vi "SCH Protection-RT Host.vi"() -> ()   [LabVIEW 2020]
doc: "Author: Scott Hannahs <sth@magnet.fsu.edu>\nCopyright 2018 Florida State University, All rights reserved."
uses:
  <vilib>/Platform/TimedLoop/XDataNode/timing_clust.ctl
  <vilib>/Platform/TimedLoop/XDataNode/nitl_modes.ctl
  <vilib>/Platform/TimedLoop/XDataNode/wakeup.ctl
  RT Server Sub VIs/RT Host Globals.vi
  <vilib>/Utility/error.llb/Error Cluster From Error Code.vi
  <vilib>/rvi/errors/niLvFpgaAdjustHostInterfaceError.vi
  <vilib>/functionblocks/Edge Detection/One Shot Falling With Input/One Shot Falling With Input.vi
  <vilib>/rvi/interface/nirviReadWriteControl/nirviReadWriteControl.xnode
  RT Controls/FPGA SCH Digitizer Ref.ctl
  <vilib>/functionblocks/FB Core/FB Core.xnode
  <vilib>/Platform/TimedLoop/XDataNode/XDataNode.xnode
  <vilib>/functionblocks/NI_FunctionBlock Libraries.lvlib
  <vilib>/NI_Real-Time Target Support.lvlib
  NiFpgaLv.dll
  <vilib>/rvi/interface/Simulation/niFpgaSimulationCallBeginRW.vi
  <vilib>/Platform/TimedLoop/XDataNode/XDNodeRunTimeDep.lvlib
panel:
  out "Finished Late?":bool
  out "Iteration Duration (microS)":i64
  in  "Data Logging Time (mS)":u32=1000
  in  "Build":u8=115
  in  "Fix":u8=2
  in  "Minor":u8=9
  in  "Major":u8=2
  out "# Network Connections":i32
  out "Error Out Connection Loop":errorcluster
  out "Mismatch":bool
  out "Error Out FIFO Loop":errorcluster
  out "#Data sets":u32
  out "Total Data Sets":u64
  out "Reading Rate":dbl format="%.1f"
  # "SCH Protection Real Time System"
  # "."
  # "."
  # "."
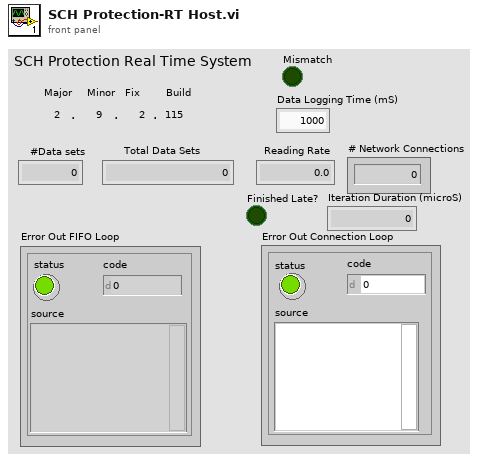
[diagram p1: front panel]
types:
  T1 = typedef "FPGA SCH Digitizer Ref.ctl" = refnum<k20>
  T2 = typedef "Net Conn Handler VI.ctl" = refnum<vi>
  T3 = typedef "XDNodeRunTimeDep.lvlib/timing_clust.ctl" = cluster{"Expected End [f-1]":u64, "Actual End [f-1]":u64, "Finished Late? [f-1]":bool, "Expected End [i-1]":u64, "Actual End [i-1]":u64, "Finished Late? [i-1]":bool, "Expected Start [i]":u64, "Actual Start [i]":u64, "Expected Start [f]":u64, "Actual Start [f]":u64, "Source Name":string, "Structure Name":string, "Period":i64, "Deadline":i64, "Offset":i64, "Start":i64, "Priority":i32, "Timeout":i32, "Mode":T4, "Wakeup Reason":T5, "Error":errorcluster, "Source Type":string, "Secondary Source Type":string, "Global End Time":u64, "Global Start Time":u64, "Frame Duration":u64, "Iteration Duration":u64, "Assigned CPU":i32, "I/O Scan Engine Mode":u32}
  T4 = typedef "XDNodeRunTimeDep.lvlib/nitl_modes.ctl" = enum32{"No Change", "Process missed periods, maintain original phase", "Discard missed periods, maintain original phase", "Process missed periods, ignore original phase", "Discard missed periods, ignore original phase"}
  T5 = typedef "XDNodeRunTimeDep.lvlib/wakeup.ctl" = enum32{"Normal", "Aborted", "Asynchronous wakeup", "Timing source error", "Timed loop error", "Timeout"}
  T6 = enum16{"Input Voltage", "Zero Voltage", "Calibrate Voltage"}
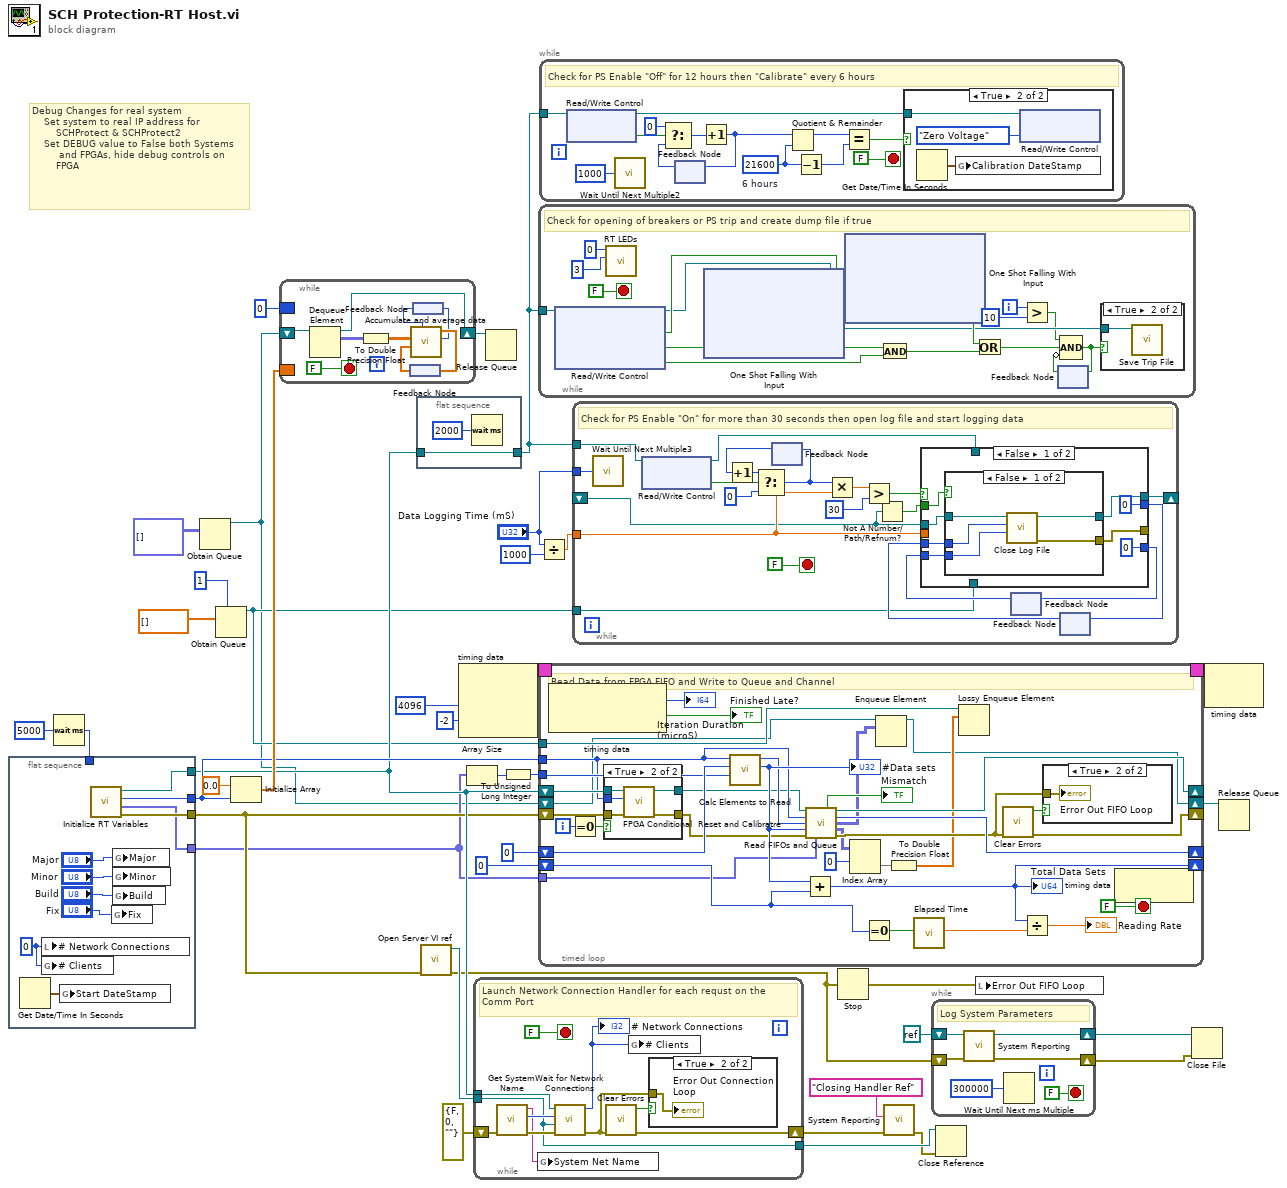
[diagram p0: block diagram]
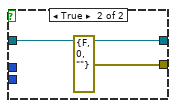
[diagram p5: hidden frame]
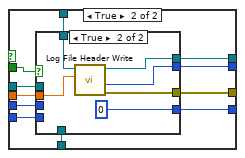
[diagram p6: hidden frame]
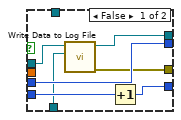
[diagram p7: hidden frame]
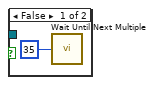
[diagram p8: hidden frame]
diagram:
  # "Debug Changes for real system\n    Set system to real IP address for\n        SCHProtect & SCHProtect2\n    Set DEBUG value to False both Systems\n         and FPGAs, hide debug controls on\n        FPGA"
  n1 = flat-sequence {
    tunnel: [w48] -> w34
    tunnel: [w47] -> w28
    tunnel: [w46] -> w30
    tunnel: w24 -> [_]
    tunnel: [w41] -> w15
    frame #0 {
      w40 = 0 ("# Connections")
      n2 = Get Date/Time In Seconds() -> (seconds since 1Jan1904=w39:timestamp)
      n3 = local write "# Network Connections"(w40) -> ()
      n4 = global write "RT Host Globals.vi" "# Clients"(w40) -> ()
      n5 = global write "RT Host Globals.vi" "Start DateStamp"(w39) -> ()
      n6 = call "Initialize RT Variables.vi"() -> ("error out"=w47:errorcluster, "Sync Guard Data"=w41:fxp<+/-,38,12>[], "Data Size"=w48:u32, "FPGA Refnum out"=w46:T1)  [unwired: 8 in]
      n7 = global write "RT Host Globals.vi" "Fix"("Fix") -> ()
      n8 = global write "RT Host Globals.vi" "Major"("Major") -> ()
      n9 = global write "RT Host Globals.vi" "Minor"("Minor") -> ()
      n10 = global write "RT Host Globals.vi" "Build"("Build") -> ()
    }
  }
  n11 = Wait (ms)(milliseconds to wait=u32 5000) -> (millisecond timer value=w24:u32)
  n12 = Obtain Queue(element data type=fxp<+/-,38,12>[][] [] ("Data Unfiltered")) -> (queue out=w3:refnum<queue>)  [unwired: 4 in, 2 out]
  n13 = Obtain Queue(max queue size (-1, unlimited)=1, element data type=dbl[] [] ("double precision float")) -> (queue out=w5:refnum<queue>)  [unwired: 3 in, 2 out]
  n14 = Initialize Array(0.0, w34) -> (w36:dbl[])
  n15 = while {
    border: w36 -> [_]
    border: 0 -> [_]
    shift-right: [w49] -> w2
    shift-left: w3 -> [w50]
    stop <- FALSE stop-if-true
    n16 = Dequeue Element(queue=w50) -> (queue out=w49:refnum<queue>, element=w51:fxp<+/-,38,12>[][])  [unwired: 2 in, 2 out]
    n17 = To Double Precision Float(number=w51) -> (double precision float=w52:dbl[][])
    n18 = feedback #1() -> (w57:dbl[])
    n19 = feedback #2() -> (w53:i32)
    n20 = call "Accumulate and average data.vi"("# Scans Accululated In"=w53, "Accumulated Array"=w57, "Raw Data In"=w52) -> ("# Scans Accumulated Out"=w54:i32, "Accumulated Array Out"=w56:dbl[])  [unwired: 7 in]
    n21 = feedback-in #1(w56) -> ()
    n22 = feedback-in #2(w54) -> ()
  }
  n23 = flat-sequence {
    tunnel: w30 -> [w59]
    tunnel: [w59] -> w33
    frame #0 {
      n24 = Wait (ms)(milliseconds to wait=u32 2000) -> ()  [unwired: 1 out]
    }
  }
  n25 = call "Open Server VI ref.vi"("error in (no error)"=w28) -> ("error out"=w12:errorcluster, "VI out"=w22:T2)  [unwired: 9 in]
  n26 = node-c288(i64 4096 ("Period"), -2 ("Processor")) -> (w17:T3)  [unwired: 1 in]
  n27 = Array Size(array=w15) -> (size(s)=w14:i32)
  n28 = while {
    shift-right: [w68] -> w20
    shift-left: errorcluster {"status"=FALSE, "code"=0, "source"=""} ("Error Out") -> [w64]
    tunnel: w30 -> [w66]
    tunnel: w22 -> [w62]
    tunnel: [w62] -> w21
    stop <- FALSE stop-if-true
    # "Launch Network Connection Handler for each requst on the Comm Port"
    n29 = call "Get System Name.vi"("Error In"=w64) -> ("Error Out"=w63:errorcluster, "Ethernet Address"=w65:u32, "System Name"=w60:string)  [unwired: 4 in]
    n30 = global write "RT Host Globals.vi" "System Net Name"(w60) -> ()
    n31 = call "Wait for Network Connections.vi"("error in (no error)"=w63, "Handler VI ref"=w62, "Ethernet Address"=w65, "FPGA Refnum in"=w66) -> ("error out"=w69:errorcluster, "# Network Connections"=w61:i32)  [unwired: 6 in]
    "# Network Connections" <- w61
    n32 = call <vilib>:"Clear Errors.vi"("error in (no error)"=w69) -> ("error out"=w68:errorcluster, "specific error cleared?"=w67:bool)  [unwired: 5 in]
    n33 = global write "RT Host Globals.vi" "# Clients"(w61) -> ()
    n34 = case shown="True" w67 {
      tunnel: w69 -> [_ w71]
      frame False {
      }
      frame True {
        "Error Out Connection Loop" <- w71
      }
    }
  }
  n35 = Release Queue(queue=w2) -> ()  [unwired: 2 in, 3 out]
  n36 = To Unsigned Long Integer(number=w14) -> (unsigned 32bit integer=w13:u32)
  n37 = while {
    tunnel: w33 -> [w87]
    i -> [w75]
    stop <- FALSE stop-if-true
    # "Check for opening of breakers or PS trip and create dump file if true"
    n38 = xnode "Read/Write Control"("FPGA VI Reference In"=w87) -> ("FPGA VI Reference Out"=w77:T1, "Breaker Enable"=w86:bool, "PS Enable"=w85:bool, "Dump File Enable"=w83:bool)  [unwired: 1 in, 1 out]
    n39 = call <vilib>:"RT LEDs.vi"("State"=3, "LED Num"=0) -> ()  [unwired: 4 in, 2 out]
    n40 = xnode "One Shot Falling With Input"("input"=w85) -> ("output"=w84:bool)  [unwired: 1 in, 1 out]
    n41 = xnode "One Shot Falling With Input"("input"=w86) -> ("output"=w82:bool)  [unwired: 1 in, 1 out]
    n42 = And(x=w84, y=w83) -> (x .and. y?=w81:bool)
    n43 = Or(x=w82, y=w81) -> (x .or. y?=w80:bool)
    n44 = Greater?(x=w75, y=10) -> (0:w76:bool)
    n45 = feedback #3() -> (w73:bool)  [unwired: 1 in]
    n46 = Compound Arithmetic op=AND(w76, w80, invert w73) -> (w72:bool)
    n47 = feedback-in #3(w72) -> ()
    n48 = case shown="True" w72 {
      tunnel: w77 -> [_ w90]
      frame False {
        n49 = call "Wait Until Next Multiple"("Count(mSec)"=u32 35) -> ()  [unwired: 1 out]
      }
      frame True {
        n50 = call "Save Trip File.vi"("FPGA Refnum"=w90) -> ()  [unwired: 10 in, 1 out]
      }
    }
  }
  n51 = Divide(x="Data Logging Time (mS)", y=u32 1000) -> (x/y=w32:dbl)
  n52 = timed-loop {
    shift-right: [w195] -> _
    shift-left: u32 0 -> [w198]
    tunnel: w34 -> [w175]
    shift-right: [w194] -> _
    shift-left: u64 0 -> [w197]
    shift-right: [w190] -> _
    shift-left: w30 -> [w178]
    shift-right: [w187] -> _
    shift-left: w28 -> [w177]
    timing: w17 -> [_]
    timing-out: [_] -> w16
    tunnel: w15 -> [w182]
    tunnel: w13 -> [w181]
    tunnel: w5 -> [w170]
    shift-right: [w167] -> w1
    shift-left: w3 -> [w168]
    i -> [w180]
    stop <- FALSE stop-if-true
    # "Read Data from FPGA FIFO and Write to Queue and Channel"
    n53 = node-c288() -> (→"Iteration Duration (microS)":i64, →"Finished Late?":bool)  [unwired: 1 in]
    n54 = Equal To 0?(x=w180) -> (x = 0?=w179:bool)
    n55 = case shown="True" w179 {
      tunnel: w178 -> [w202 w207]
      tunnel: [w202 w206] -> w172
      tunnel: [w201 w205] -> w176
      tunnel: w177 -> [w201 w204]
      tunnel: w175 -> [_ w203]
      frame False {
      }
      frame True {
        n56 = call "FPGA Conditional  Reset and Calibratre.vi"("error in (no error)"=w204, "Data Size"=w203, "Refnum in"=w207) -> ("error out"=w205:errorcluster, "Refnum out"=w206:T1)  [unwired: 6 in, 1 out]
      }
    }
    n57 = call "Calc Elements to Read.vi"("Sync Guard Data Length"=w181, "Elements in FIFO"=w198, "Data Size"=w175) -> ("# Data Sets To Read"=w192:u32, "# Elements to Read"=w188:u32)  [unwired: 7 in]
    "#Data sets" <- w192
    n58 = Add(x=w192, y=w197) -> (x+y=w194:u64)
    "Total Data Sets" <- w194
    n59 = call "Read FIFOs and Queue.vi"("FPGA VI Reference"=w172, "Data Size"=w175, "# Elements to Read"=w188, "# Data Sets To Read"=w192, "error in (no error)"=w176, "Sync Guard Data"=w182) -> ("Read Mismatch"=→"Mismatch":bool, "Refnum out"=w190:T1, "Elements Remaining"=w195:u32, "Data Unfiltered"=w169:fxp<+/-,38,12>[][], "DataFiltered"=w184:fxp<+/-,38,12>[][], "error out"=w189:errorcluster)  [unwired: 4 in]
    n60 = Index Array(array=w184, index (row)=0 ("index")) -> (element=w183:fxp<+/-,38,12>[])  [unwired: 1 in]
    n61 = Equal To 0?(x=w197) -> (x = 0?=w199:bool)
    n62 = Enqueue Element(queue=w168, element=w169) -> (queue out=w167:refnum<queue>)  [unwired: 2 in, 2 out]
    n63 = To Double Precision Float(number=w183) -> (double precision float=w171:dbl[])
    n64 = call "Elapsed Time"("Reset"=w199) -> ("Elapsed Time (s)"=w200:dbl)  [unwired: 11 in, 7 out]
    n65 = Lossy Enqueue Element(queue=w170, element=w171) -> ()  [unwired: 1 in, 4 out]
    n66 = call <vilib>:"Clear Errors.vi"("error in (no error)"=w189) -> ("error out"=w187:errorcluster, "specific error cleared?"=w186:bool)  [unwired: 5 in]
    n67 = Divide(x=w194, y=w200) -> (x/y=→"Reading Rate":dbl)
    n68 = case shown="True" w186 {
      tunnel: w189 -> [_ w212]
      frame False {
      }
      frame True {
        "Error Out FIFO Loop" <- w212
      }
    }
    n69 = node-c288() -> ()  [unwired: 1 in, 1 out]
  }
  n70 = while {
    tunnel: w33 -> [w224]
    stop <- FALSE stop-if-true
    w216 = 21600  # 6 hours
    # "Check for PS Enable \"Off\" for 12 hours then \"Calibrate\" every 6 hours"
    n71 = xnode "Read/Write Control"("FPGA VI Reference In"=w224) -> ("FPGA VI Reference Out"=w220:T1, "PS Enable"=w218:bool)  [unwired: 1 in, 1 out]
    n72 = call "Wait Until Next Multiple2"("Count(mSec)"=u32 1000) -> ()  [unwired: 1 out]
    n73 = feedback #4() -> (w219:i32)  [unwired: 1 in]
    n74 = Select(t=0 ("y"), s=w218, f=w219) -> (s? t:f=w223:i32)
    n75 = Increment(x=w223) -> (x+1=w221:i32)
    n76 = feedback-in #4(w221) -> ()
    n77 = Quotient & Remainder(x=w221, y=w216) -> (x-y*floor(x/y)=w217:i32)  [unwired: 1 out]
    n78 = Decrement(x=w216) -> (x-1=w215:i32)
    n79 = Equal?(x=w217, y=w215) -> (x = y?=w214:bool)
    n80 = case shown="True" w214 {
      tunnel: w220 -> [_ w227]
      frame False {
      }
      frame True {
        n81 = Get Date/Time In Seconds() -> (seconds since 1Jan1904=w226:timestamp)
        n82 = global write "RT Host Globals.vi" "Calibration DateStamp"(w226) -> ()
        n83 = xnode "Read/Write Control"("FPGA VI Reference In"=w227, "Input Select"=T6."Zero Voltage") -> ()  [unwired: 1 in, 2 out]
      }
    }
  }
  n84 = while {
    tunnel: w33 -> [w248]
    tunnel: w32 -> [w240]
    shift-right: [w236] -> _
    shift-left: _ -> [w239]
    tunnel: "Data Logging Time (mS)" -> [w230]
    tunnel: w5 -> [w229]
    stop <- FALSE stop-if-true
    # "Check for PS Enable \"On\" for more than 30 seconds then open log file and start logging data"
    n85 = call "Wait Until Next Multiple3"("Count(mSec)"=w230) -> ()  [unwired: 1 out]
    n86 = xnode "Read/Write Control"("FPGA VI Reference In"=w248) -> ("FPGA VI Reference Out"=w231:T1, "PS Enable"=w247:bool)  [unwired: 1 in, 1 out]
    n87 = feedback #5() -> (w245:i32)  [unwired: 1 in]
    n88 = Increment(x=w245) -> (x+1=w243:i32)
    n89 = Select(t=w243, s=w247, f=0 ("y")) -> (s? t:f=w244:i32)
    n90 = feedback-in #5(w244) -> ()
    n91 = Multiply(x=w244, y=w240) -> (x*y=w242:dbl)
    n92 = Greater?(x=w242, y=30) -> (0:w238:bool)
    n93 = Not A Number/Path/Refnum?(number/path/refnum=w239) -> (NaN/Path/Refnum?=w237:bool)
    n94 = feedback #6() -> (w232:i32)  [unwired: 1 in]
    n95 = feedback #7() -> (w234:i64)  [unwired: 1 in]
    n96 = case shown="False" w238 {
      tunnel: w240 -> [_ w275]
      tunnel: [w255 w274] -> w236
      tunnel: w239 -> [w256 w267]
      tunnel: [w252 w273] -> _
      tunnel: w237 -> [w257 w272]
      tunnel: w234 -> [w254 w268]
      tunnel: [i64 0 ("offset for # rows") w271] -> w235
      tunnel: w232 -> [w253 w269]
      tunnel: [0 w270] -> w233
      tunnel: w229 -> [_ w266]
      tunnel: w231 -> [_ w265]
      frame False {
        n97 = case shown="False" w257 {
          tunnel: w256 -> [w262 w264]
          tunnel: [w261 w264] -> w255
          tunnel: [w260 errorcluster {"status"=FALSE, "code"=0, "source"=""} ("Error Out")] -> w252
          tunnel: w254 -> [w259 _]
          tunnel: w253 -> [w258 _]
          frame False {
            n98 = call "Close Log File.vi"("# Rows"=w258, "Offset # Rows"=w259, "Byte Stream File in"=w262) -> ("Error Out"=w260:errorcluster, "Byte Stream File out"=w261:refnum<file>)  [unwired: 7 in]
          }
          frame True {
          }
        }
      }
      frame True {
        n99 = case shown="True" w272 {
          tunnel: w275 -> [_ w288]
          tunnel: [w278 w287] -> w274
          tunnel: [w277 w286] -> w273
          tunnel: [w280 w285] -> w271
          tunnel: [w281 0] -> w270
          tunnel: w269 -> [w282 _]
          tunnel: w268 -> [w280 _]
          tunnel: w267 -> [w279 _]
          tunnel: w266 -> [w276 _]
          tunnel: w265 -> [_ w283]
          frame False {
            n100 = call "Write Data to Log File.vi"("queue out"=w276, "Byte Stream File in"=w279) -> ("error out"=w277:errorcluster, "Byte Stream File out"=w278:refnum<file>)  [unwired: 8 in]
            n101 = Increment(x=w282) -> (x+1=w281:i32)
          }
          frame True {
            n102 = call "Log File Header Write.vi"("Raw Data Period"=w288, "FPGA Refnum"=w283) -> ("error out"=w286:errorcluster, "offset for # rows"=w285:i64, "Byte Stream File out"=w287:refnum<file>)  [unwired: 6 in, 1 out]
          }
        }
      }
    }
    n103 = feedback-in #6(w233) -> ()
    n104 = feedback-in #7(w235) -> ()
  }
  n105 = Stop(stop? (T)=w12) -> ()
  n106 = call "System Reporting.vi"("Error In"=w20, "String"="Closing Handler Ref") -> ("Error Out"=w19:errorcluster)  [unwired: 8 in, 1 out]
  n107 = while {
    shift-right: [w292] -> w27
    shift-left: refnum<k0> refnum ("Byte Stream File out") -> [w293]
    shift-right: [w289] -> w25
    shift-left: w12 -> [w290]
    stop <- FALSE stop-if-true
    # "Log System Parameters"
    n108 = call "System Reporting.vi"("Error In"=w290, "Byte Stream File in"=w293) -> ("Error Out"=w289:errorcluster, "Byte Stream File out"=w292:refnum<file>)  [unwired: 8 in]
    n109 = Wait Until Next ms Multiple(millisecond multiple=u32 300000) -> ()  [unwired: 1 out]
  }
  n110 = Close Reference(reference=w21, error in (no error)=w19) -> ()  [unwired: 1 out]
  n111 = local write "Error Out FIFO Loop"(w12) -> ()
  n112 = Close File(refnum=w27, error in=w25) -> ()  [unwired: 2 out]
  n113 = node-c288(w16) -> ()  [unwired: 1 out]
  n114 = Release Queue(queue=w1) -> ()  [unwired: 2 in, 3 out]
